vi "RTS Build Point File Data.vi"(4 "Force Read Point?":bool, 6 "Disable System Time Filter":bool, 8 "Error In":errorcluster, 10 "Full List Box Data":string[][](array[string]), 11 "Point File Location":path) -> (0 "Error Out":errorcluster, 1 "Custom Titles":string[](array[string]), 2 "Custom Listbox Data":string[][](array[string]), 3 "Point File":T1[](array[typedef]))   [LabVIEW 2018]
uses:
  Type Definitions/RTS Point File.ctl
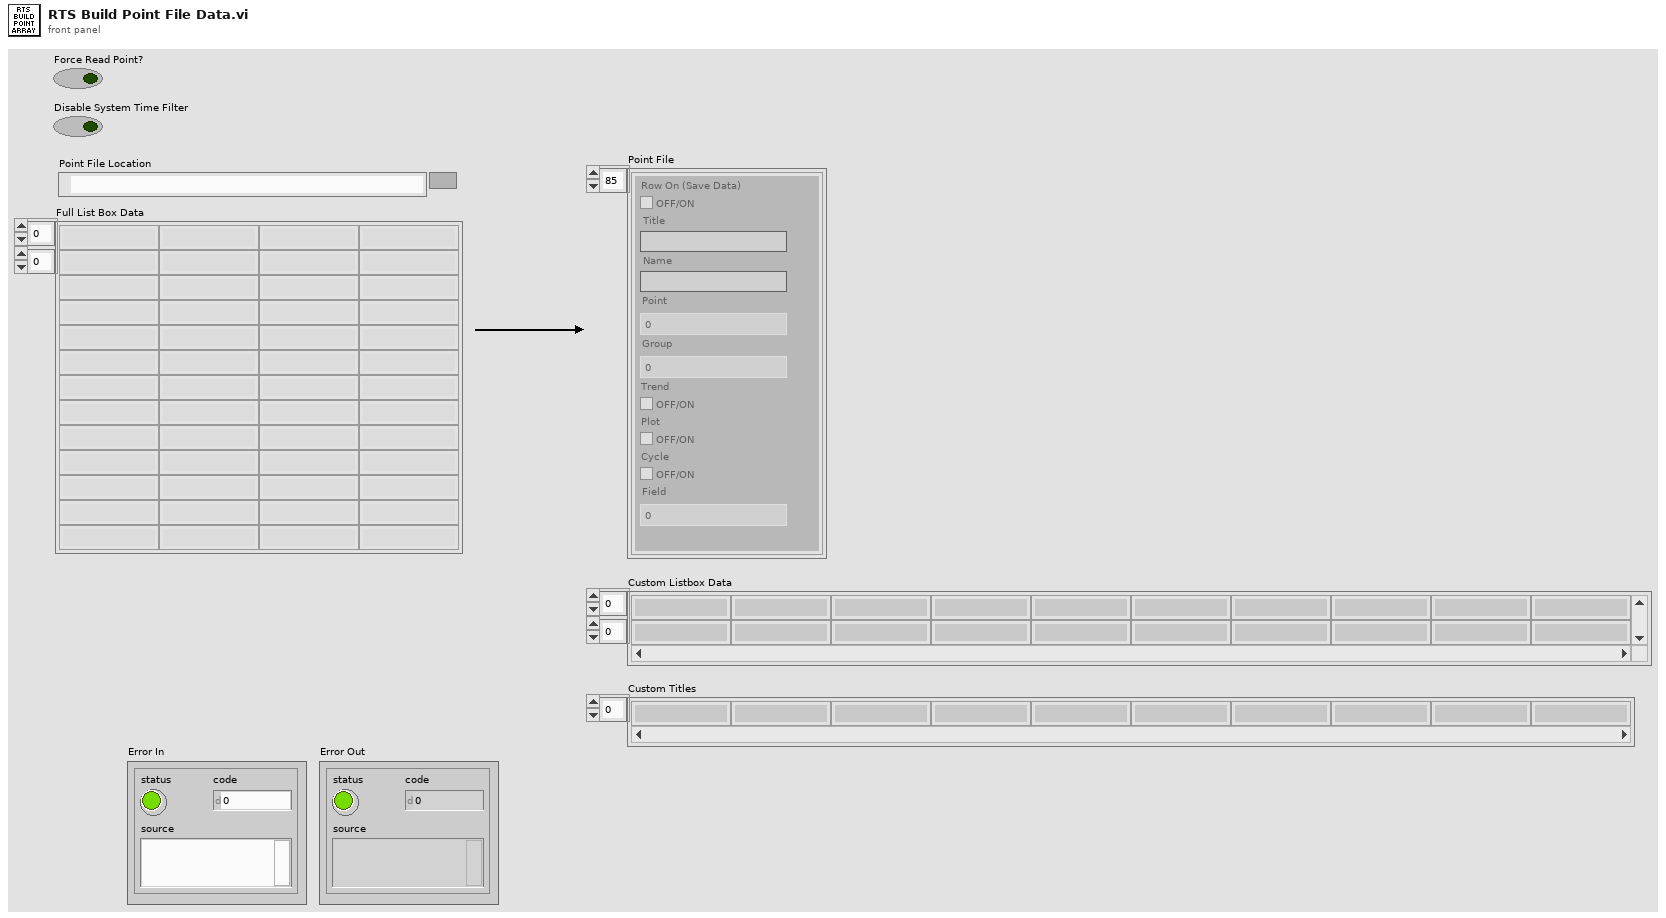
[diagram p1: front panel]
types:
  T1 = typedef "RTS Point File.ctl" = cluster{"Title":string, "Name":string, "Point":u8, "Plot":bool, "Trend":bool, "Cycle":bool, "Field":u8, "Row On (Save Data)":bool, "Group":u8}
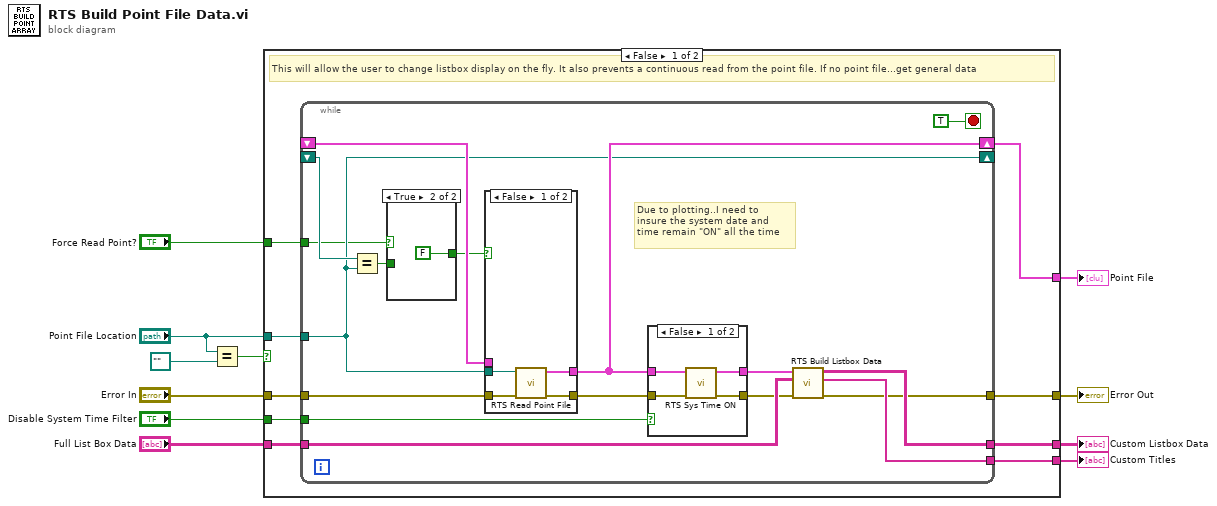
[diagram p0: block diagram]
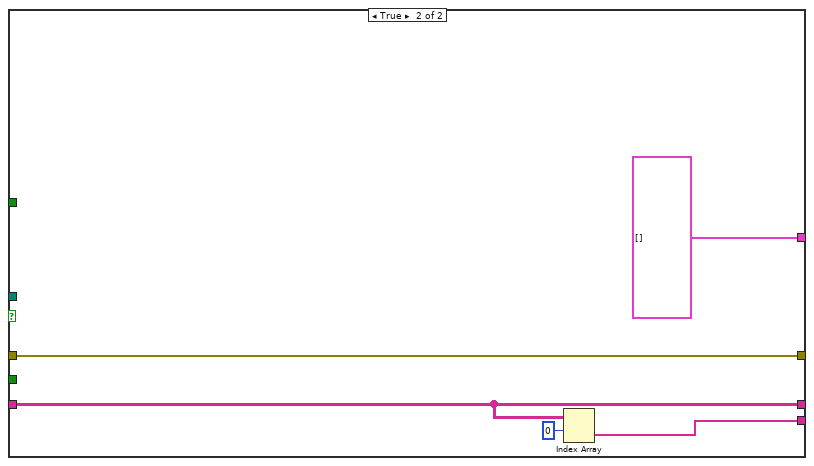
[diagram p5: hidden frame]
diagram:
  n1 = Equal?(x="Point File Location", y=path "") -> (x = y?=w6:bool)
  n2 = case shown="False" w6 {
    tunnel: [w20 w55] -> w10
    tunnel: "Point File Location" -> [w18 _]
    tunnel: "Full List Box Data" -> [w19 w55]
    tunnel: [w17 T1[] [] ("Point File")] -> w9
    tunnel: [w16 w53] -> w11
    tunnel: "Error In" -> [w15 w52]
    tunnel: [w14 w52] -> w3
    tunnel: "Disable System Time Filter" -> [w13 _]
    tunnel: "Force Read Point?" -> [w12 _]
    frame False {
      # "This will allow the user to change listbox display on the fly. It also prevents a continuous read from the point file. If no point file...get general data"
      n3 = while {
        shift-right: [w28] -> _
        shift-left: _ -> [w31]
        tunnel: w18 -> [w28]
        shift-right: [w30] -> w17
        shift-left: _ -> [w29]
        tunnel: w19 -> [w35]
        tunnel: [w36] -> w20
        tunnel: [w27] -> w16
        tunnel: w15 -> [w26]
        tunnel: [w25] -> w14
        tunnel: w13 -> [w24]
        tunnel: w12 -> [w23]
        stop <- TRUE stop-if-true
        # "Due to plotting..I need to\ninsure the system date and\ntime remain \"ON\" all the time"
        n4 = Equal?(x=w31, y=w28) -> (x = y?=w21:bool)
        n5 = case shown="True" w23 {
          tunnel: [w38 FALSE] -> w22
          tunnel: w21 -> [w38 _]
          frame False {
          }
          frame True {
          }
        }
        n6 = case shown="False" w22 {
          tunnel: [w49 w51] -> w30
          tunnel: [w48 w50] -> w34
          tunnel: w29 -> [_ w51]
          tunnel: w26 -> [w47 w50]
          tunnel: w28 -> [w46 _]
          frame False {
            n7 = call "RTS Read Point File.vi"("Error In"=w47, "Path"=w46) -> ("Error Out"=w48:errorcluster, "Point File"=w49:T1[])  [unwired: 7 in, 1 out]
          }
          frame True {
          }
        }
        n8 = case shown="False" w24 {
          tunnel: [w43 w44] -> w37
          tunnel: w34 -> [w42 w45]
          tunnel: [w41 w45] -> w33
          tunnel: w30 -> [w40 w44]
          frame False {
            n9 = call "RTS Sys Time ON.vi"("Error In"=w42, "Point File in"=w40) -> ("Error Out"=w41:errorcluster, "Point File out"=w43:T1[])  [unwired: 8 in]
          }
          frame True {
          }
        }
        n10 = call "RTS Build Listbox Data.vi"("Error In"=w33, "Full Data Set Input"=w35, "Point File in"=w37) -> ("Error Out"=w25:errorcluster, "Custom Titles"=w27:string[], "Custom Listbox Data"=w36:string[][])  [unwired: 6 in]
      }
    }
    frame True {
      n11 = Index Array(array=w55, index (row)=0) -> (element=w53:string[])  [unwired: 1 in]
    }
  }
  "Custom Listbox Data" <- w10
  "Point File" <- w9
  "Custom Titles" <- w11
  "Error Out" <- w3
